vi "Remove Key-Value Pair.vi"(8 "error in (no error)":errorcluster, 10 "key":string, 11 "URI-Component.Query in":refnum<class "URI-Component.Query.lvclass">) -> (0 "error out":errorcluster, 1 "deleted":bool, 3 "URI-Component.Query":refnum<class "URI-Component.Query.lvclass">)   [LabVIEW 2013, in "openURI.lvlib" / "URI-Component.Query.lvclass"]
uses:
  URI-Component.Query.lvclass
  URI-Component.Query.lvclass/URI-Component.Query.ctl
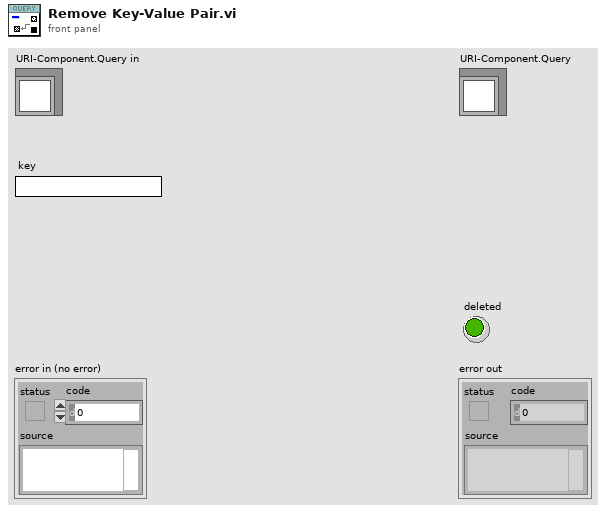
[diagram p1: front panel]
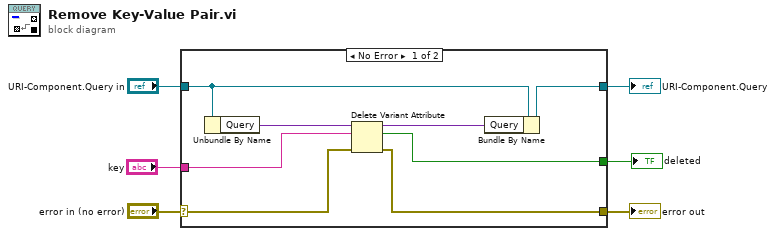
[diagram p0: block diagram]
diagram:
  n1 = case shown="No Error" "error in (no error)" {
    selector: "error in (no error)" -> [w8 w15]
    tunnel: [w7 w15] -> w5
    tunnel: [w13 w16] -> w3
    tunnel: "URI-Component.Query in" -> [w14 w16]
    tunnel: "key" -> [w11 _]
    tunnel: [w10 _] -> w1
    frame No Error {
      n2 = Unbundle By Name(w14) -> ("Query"=w12:variant)
      n3 = Delete Variant Attribute(4:w8, 6:w11, 7:w12) -> (0:w7:errorcluster, 2:w10:bool, 3:w9:variant)
      n4 = Bundle By Name(cluster=w14, "Query"=w9) -> (w13:refnum<class "URI-Component.Query.lvclass">)
    }
    frame Error {
    }
  }
  "error out" <- w5
  "URI-Component.Query" <- w3
  "deleted" <- w1
